vi "changeColorStatus.vi"(11 "Enum in":refnum<vi>) -> ()   [LabVIEW 2013]
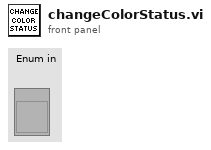
[diagram p1: front panel]
types:
  T1 = typedef "TRAServer.lvclass/StatusTRA_TypDef.ctl" = enum16{"NOT REFERENCED", "CONFIGURATION", "HOMING", "MOVING", "READY", "DISABLE", "JOGGING"}
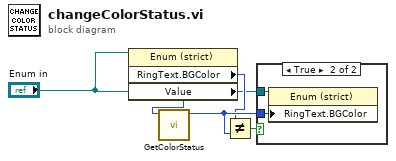
[diagram p0: block diagram]
diagram:
  n1 = property class="Enum (strict)"(reference="Enum in") -> ("RingText.BGColor"=w2:u32, "Value"=w5:T1)  [unwired: 1 in, 2 out]
  n2 = call "GetColorStatus.vi"("Status"=w5) -> ("Numeric"=w3:u32)  [unwired: 10 in]
  n3 = Not Equal?(x=w2, y=w3) -> (x != y?=w4:bool)
  n4 = case shown="True" w4 {
    tunnel: "Enum in" -> [_ w7]
    tunnel: w3 -> [_ w6]
    frame False {
    }
    frame True {
      n5 = property class="Enum (strict)"(reference=w7, "RingText.BGColor"=w6) -> ()  [unwired: 1 in, 2 out]
    }
  }
